vi "M100DailyOutputAutoNew.vi"() -> ()   [LabVIEW 2012]
uses:
  <vilib>/Utility/NIReport.llb/NI_report.lvclass
  <vilib>/addons/database/Connection.llb/DB Tools Open Connec (Path).vi
  <vilib>/addons/database/Connection.llb/Conn Execute.vi
  <vilib>/addons/database/Recordset.llb/Rec Fetch Recordset Data (R).vi
  <vilib>/addons/database/Recordset.llb/Rec Destroy - Connection.vi
  <vilib>/Utility/NIReport.llb/Append Text Table to Report (wrap).vi
  <vilib>/addons/database/_DB Variant To Data/Database Variant To Data.xnode
  <vilib>/addons/database/NI_Database_API.lvlib
  <vilib>/Utility/SMTP/NI_SMTPEmail.lvlib
  <vilib>/Utility/NIReport.llb/Excel/NI_Excel.lvclass
  <vilib>/addons/_office/NI_ReportGenerationToolkit.lvlib
panel:
  in  "Table Control 3":string[][](table)
  out "error out 4":errorcluster
  in  "Table Control 2":string[][](table)
  out "error out 3":errorcluster
  in  "Table Control":string[][](table)
  out "error out 2":errorcluster
  in  "Report Template":path=path "O:/Monitor/Report/M100DailyOutput.xls"
  out "error out":errorcluster
  out "spreadsheet string":string
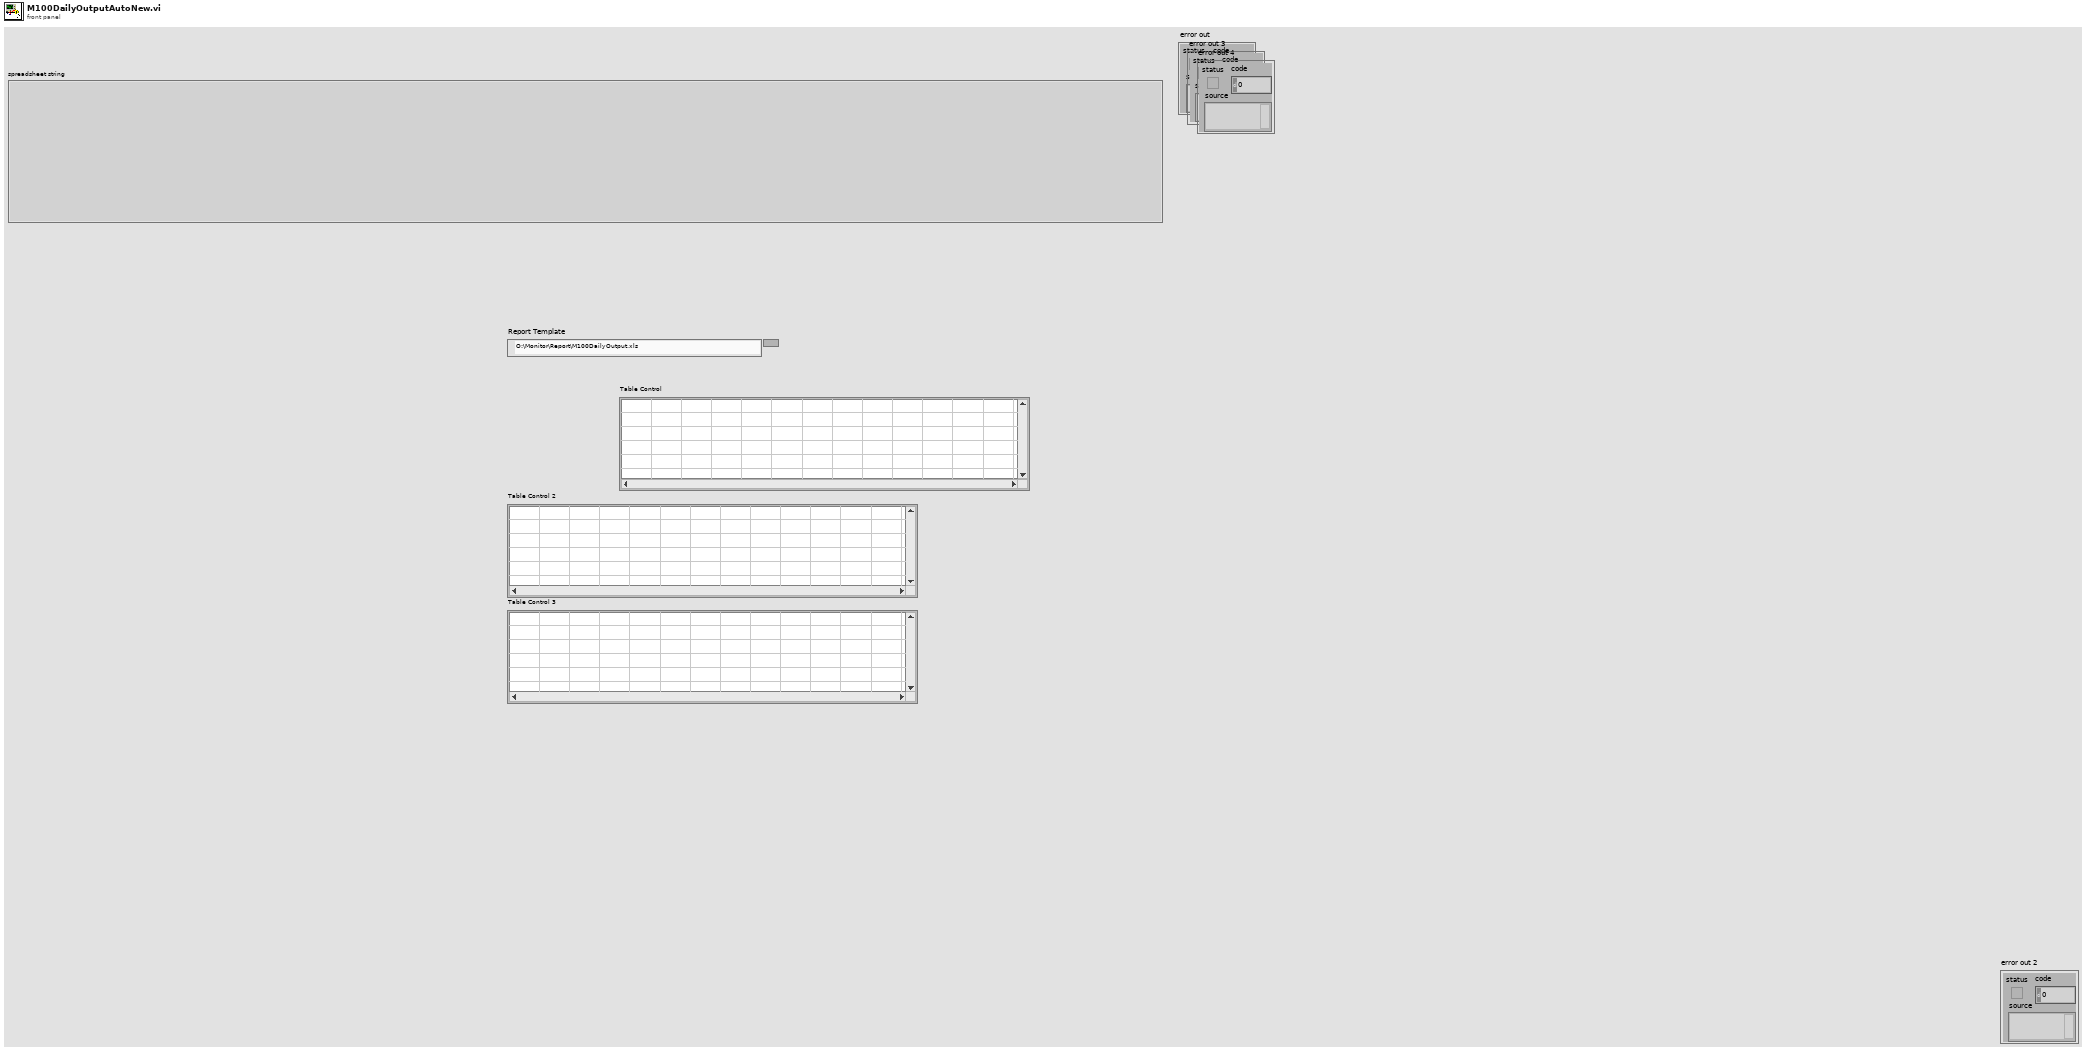
[diagram p1: front panel]
types:
  T1 = typedef "NI_Database_API.lvlib/Conn ObjectReference.ctl" = refnum<k1>
  T2 = typedef "NI_Database_API.lvlib/Rec ObjectReference.ctl" = refnum<k1>
  T3 = enum16{"Standard Report", "HTML", "Word", "Excel"}
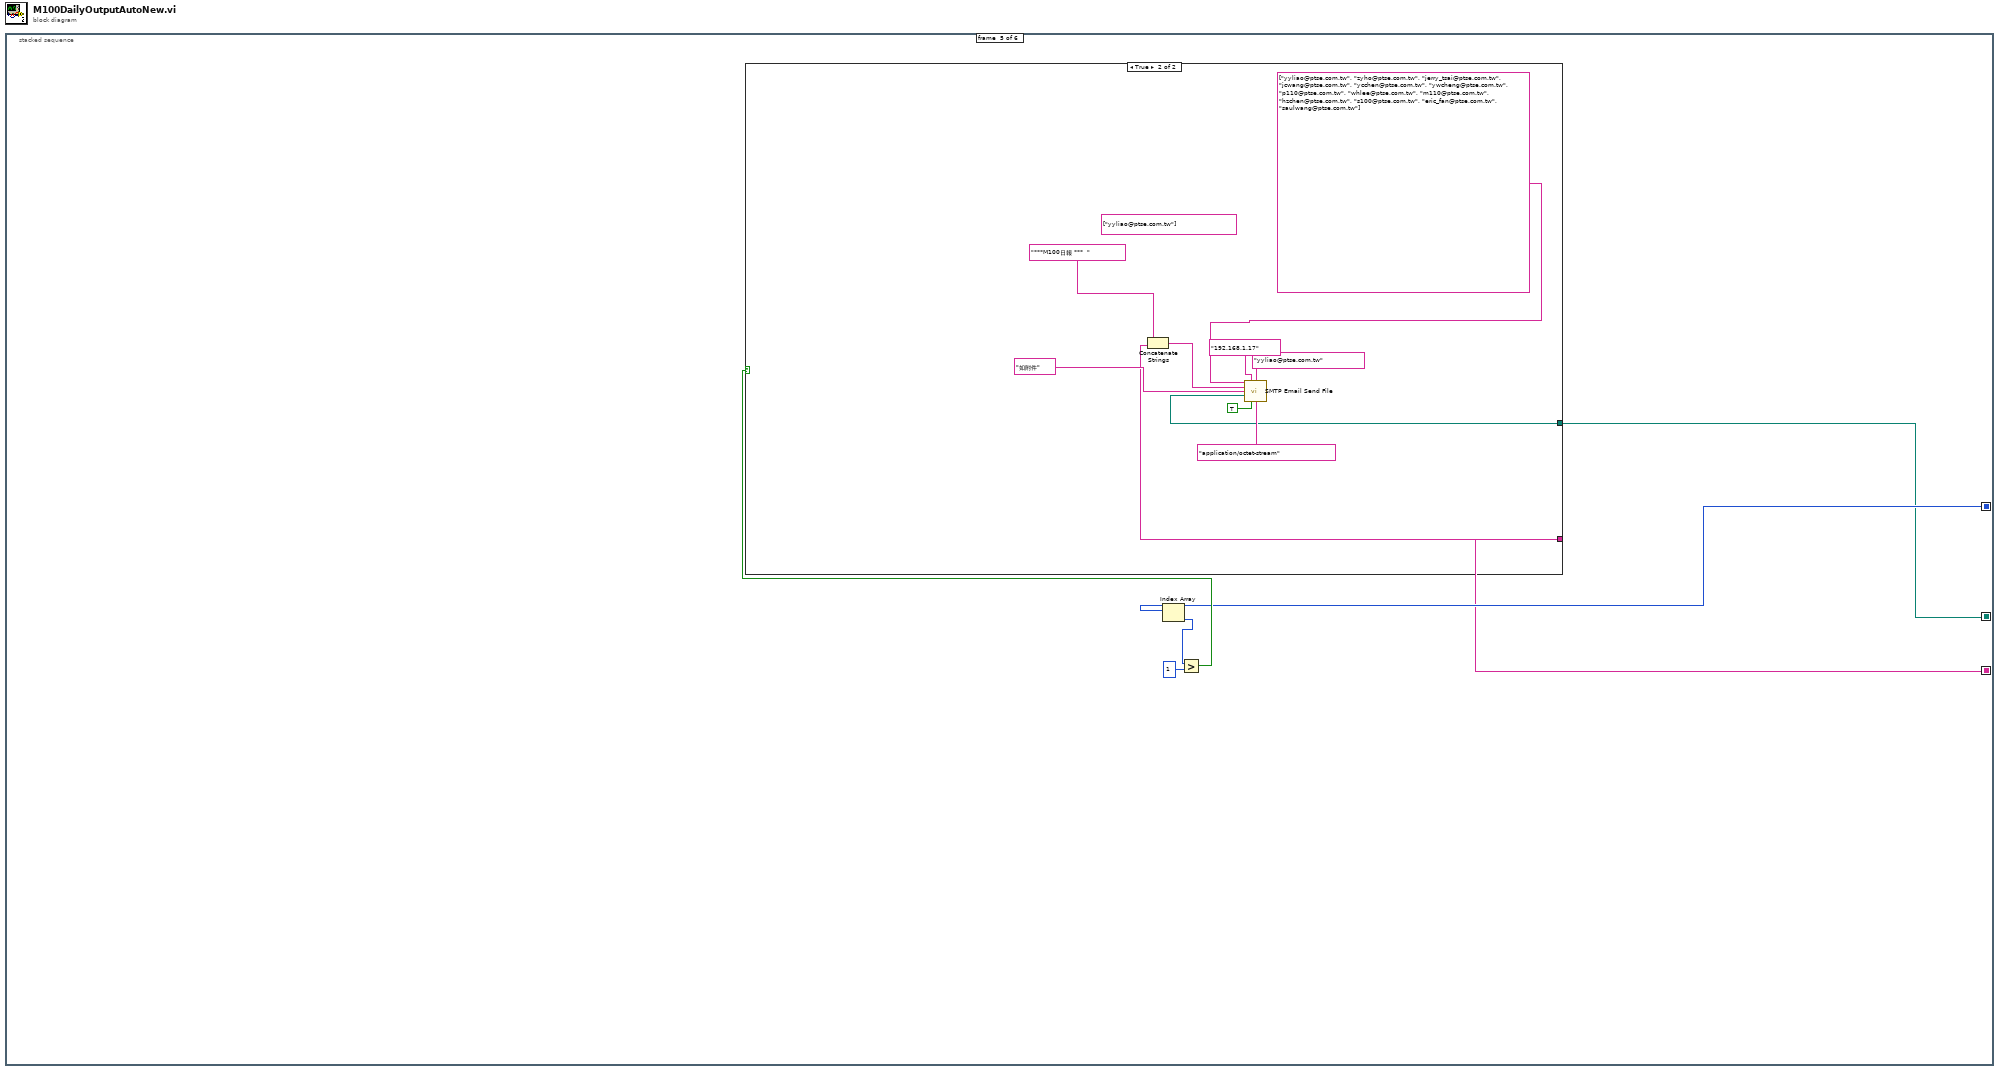
[diagram p0: block diagram]
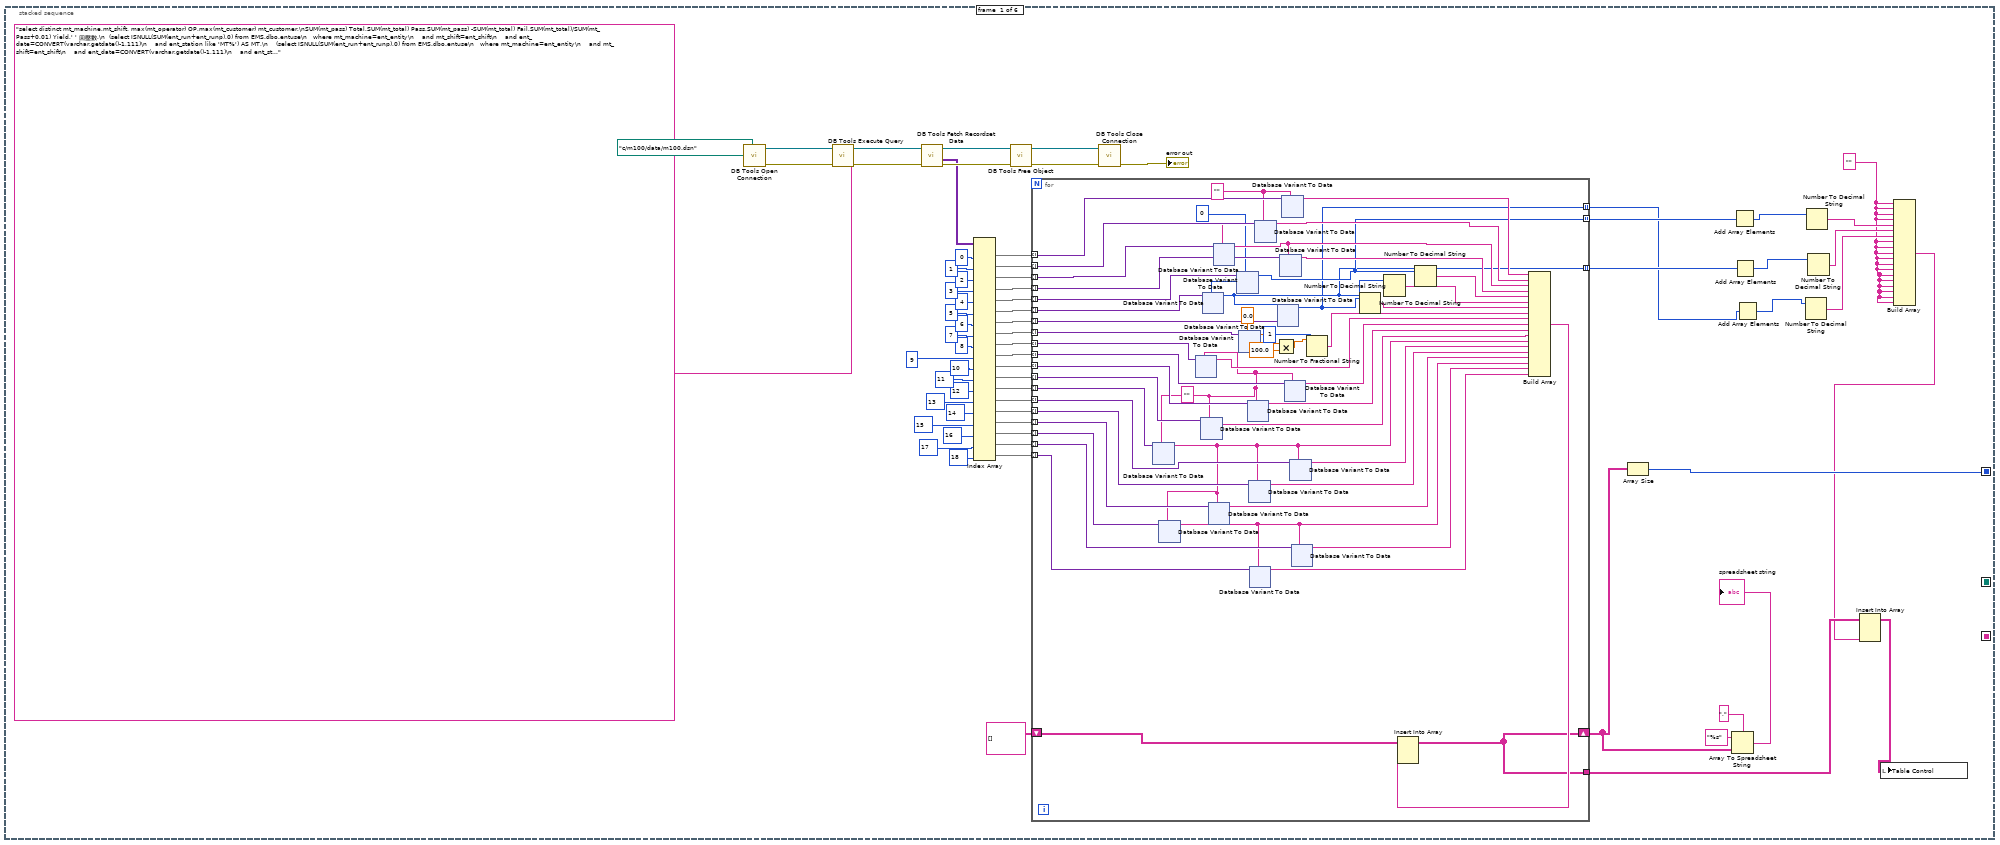
[diagram p2: hidden frame]
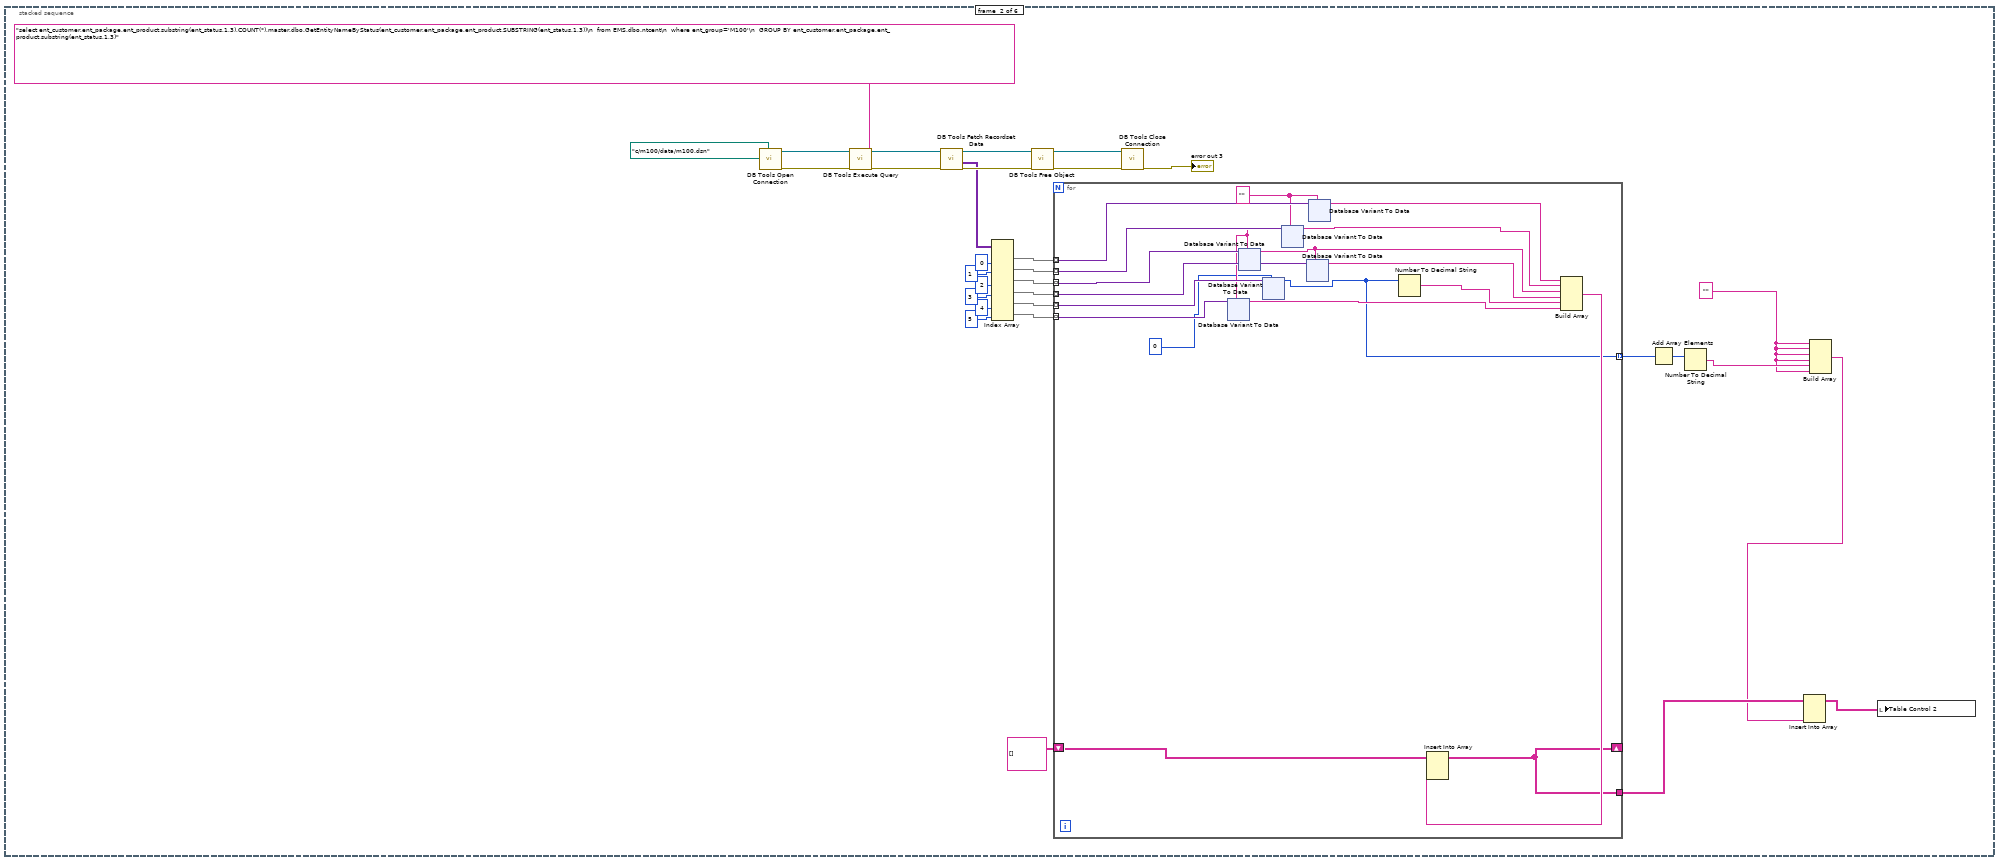
[diagram p3: hidden frame]
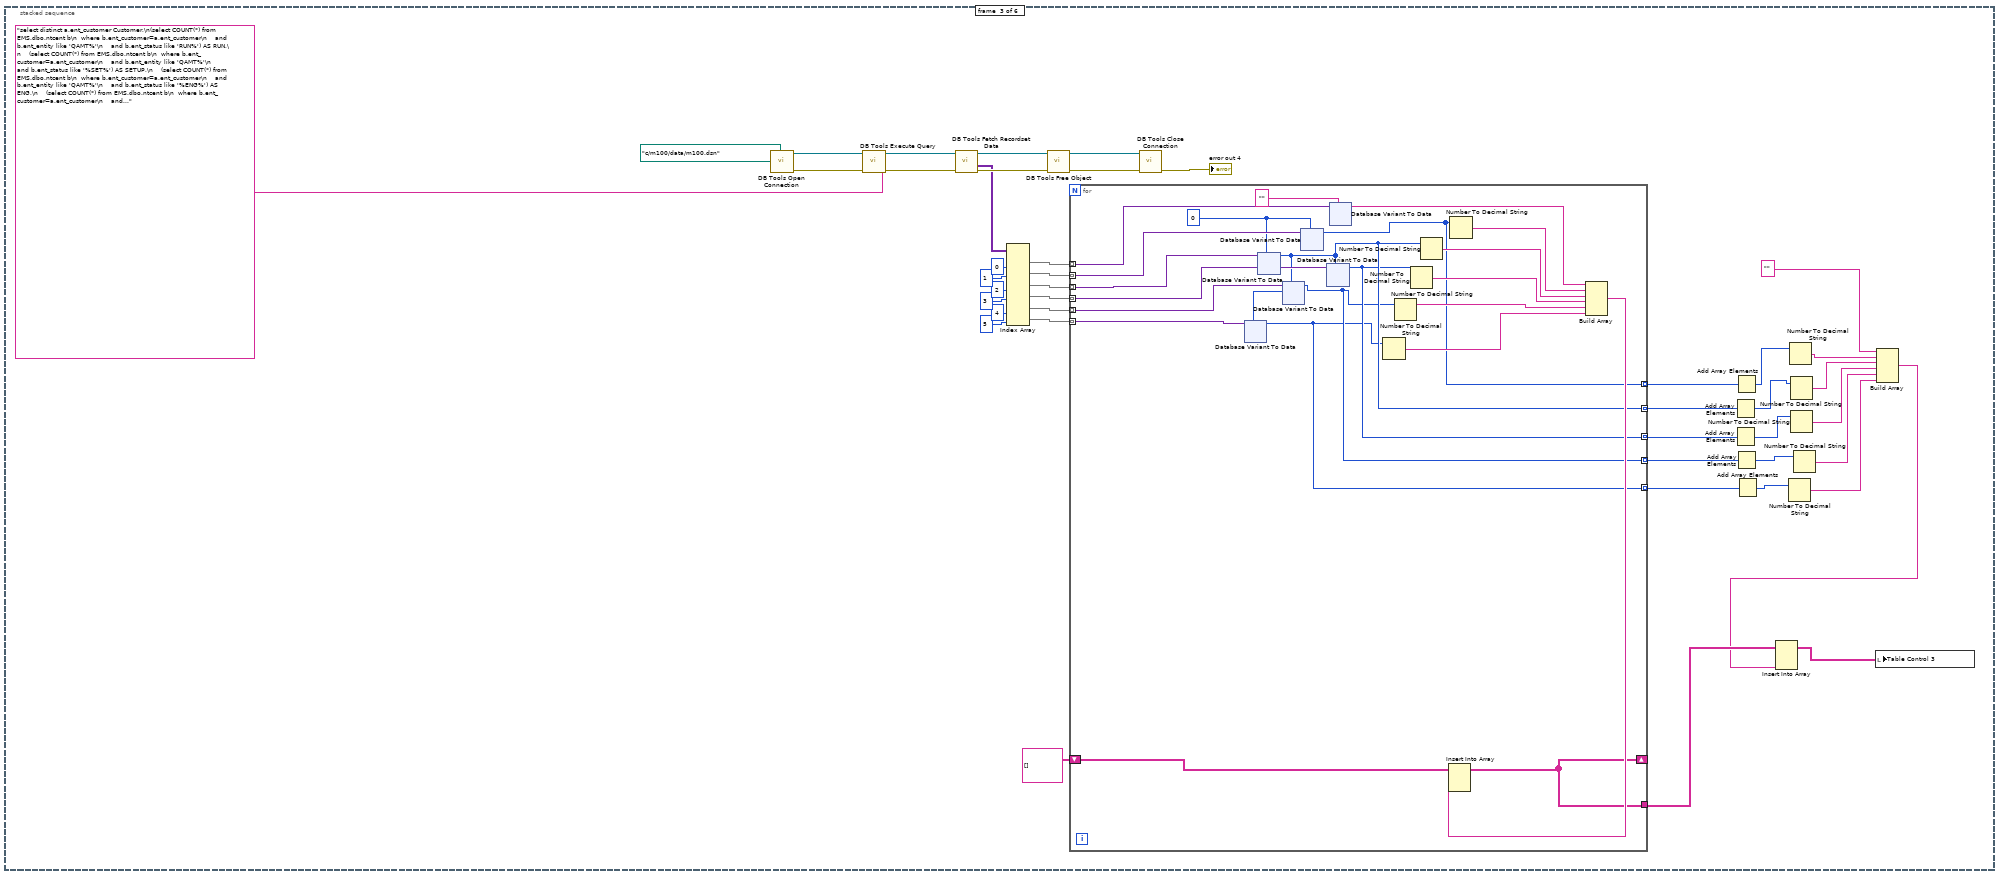
[diagram p4: hidden frame]
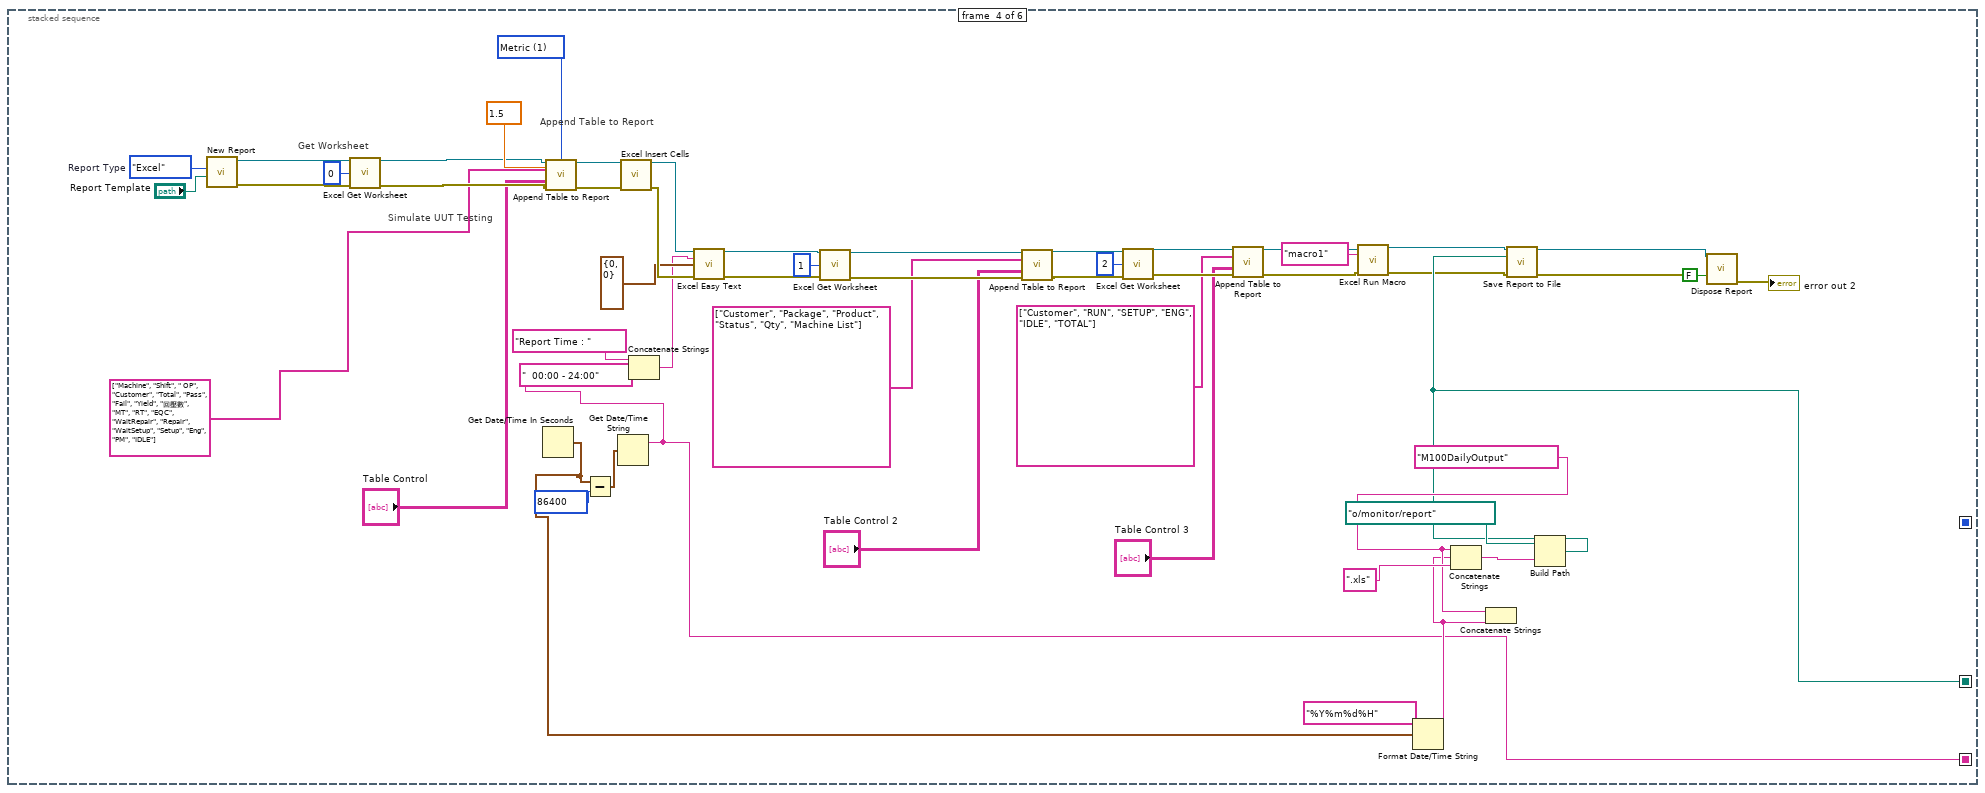
[diagram p5: hidden frame]
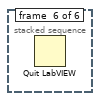
[diagram p7: hidden frame]
diagram:
  n1 = stacked-sequence {
    seq-local: [w37 _ _ _ _ _] -> [_ _ _ _ w1285 _]
    seq-local: [_ _ _ w1251 _ _] -> [_ _ _ _ w1284 _]
    seq-local: [_ _ _ w1250 _ _] -> [_ _ _ _ w1283 _]
    frame #0 {
      w4 = ""
      n2 = call-poly <vilib>:"DB Tools Open Connection.vi"("connection information"=path "c:/m100/data/m100.dsn") -> ("error out"=w64:errorcluster, "connection reference"=w68:T1)  [unwired: 7 in]
      n3 = call-poly <vilib>:"DB Tools Execute Query.vi"("error in (no error)"=w64, "SQL query"="select distinct mt_machine,mt_shift, max(mt_operator) OP,max(mt_customer) mt_customer,\nSUM(mt_pass) Total,SUM(mt_total) Pass,SUM(mt_pass) -SUM(mt_total) Fail,SUM(mt_total)/SUM(mt_Pass+0.01) Yield,' ' 回壓數,\n  (select ISNULL(SUM(ent_run+ent_runp),0) from EMS.dbo.entuse\n   where mt_machine=ent_entity\n    and mt_shift=ent_shift\n    and ent_date=CONVERT(varchar,getdate()-1,111)\n    and ent_station like 'MT%') AS MT,\n    (select ISNULL(SUM(ent_run+ent_runp),0) from EMS.dbo.entuse\n   where mt_machine=ent_entity\n    and mt_shift=ent_shift\n    and ent_date=CONVERT(varchar,getdate()-1,111)\n    and ent_station like 'RT%') AS RT,\n    (select ISNULL(SUM(ent_run+ent_runp),0) from EMS.dbo.entuse\n   where mt_machine=ent_entity\n    and mt_shift=ent_shift\n    and ent_date=CONVERT(varchar,getdate()-1,111)\n    and ent_station like 'EQ%') AS EQC,\n    (select ISNULL(SUM(ent_wait_repair),0) from EMS.dbo.entuse\n   where mt_machine=ent_entity\n    and mt_shift=ent_shift\n    and ent_date=CONVERT(varchar,getdate()-1,111)) as WaitRepair,\n     (select ISNULL(SUM(ent_repair),0) from EMS.dbo.entuse\n   where mt_machine=ent_entity\n    and mt_shift=ent_shift\n    and ent_date=CONVERT(varchar,getdate()-1,111)) as Repair,\n    (select ISNULL(SUM(ent_wait_setup),0) from EMS.dbo.entuse\n   where mt_machine=ent_entity\n    and mt_shift=ent_shift\n    and ent_date=CONVERT(varchar,getdate()-1,111)) as WaitSetup,\n     (select ISNULL(SUM(ent_setup),0) from EMS.dbo.entuse\n   where mt_machine=ent_entity\n    and mt_shift=ent_shift\n    and ent_date=CONVERT(varchar,getdate()-1,111)) as Setup,\n    (select ISNULL(SUM(ent_eng),0) from EMS.dbo.entuse\n   where mt_machine=ent_entity\n    and mt_shift=ent_shift\n    and ent_date=CONVERT(varchar,getdate()-1,111)) as Eng,\n     (select ISNULL(SUM(ent_pm),0) from EMS.dbo.entuse\n   where mt_machine=ent_entity\n    and mt_shift=ent_shift\n    and ent_date=CONVERT(varchar,getdate()-1,111)) as PM,\n    (select ISNULL(SUM(ent_idle),0) from EMS.dbo.entuse\n   where mt_machine=ent_entity\n    and mt_shift=ent_shift\n    and ent_date=CONVERT(varchar,getdate()-1,111)) as IDLE\n  from m100.dbo.mt_data\n  where CONVERT(varchar,mt_end,111)=CONVERT(varchar,getdate()-1,111)\n    and mt_machine like 'QAMT%'\n  group by mt_machine,mt_shift\n  order by mt_machine,mt_shift desc", "connection reference"=w68) -> ("error out"=w63:errorcluster, "recordset reference"=w67:T2)  [unwired: 5 in]
      n4 = call-poly <vilib>:"DB Tools Fetch Recordset Data.vi"("error in (no error)"=w63, "recordset reference"=w67) -> ("error out"=w62:errorcluster, "recordset data"=w31:variant[][], "recordset reference out"=w66:T2)  [unwired: 3 in]
      n5 = Index Array(array=w31, index (col) #1=0 ("disabled index (col)"), index (col) #2=1 ("index (col)"), index (col) #3=2 ("index (col)"), index (col) #4=3 ("index (col)"), index (col) #5=4 ("index (col)"), index (col) #6=5 ("index (col)"), index (col) #7=6 ("index (col)"), index (col) #8=7 ("index (col)"), index (col) #9=8 ("index (col)"), index (col) #10=9 ("index (col)"), index (col) #11=10 ("index (col)"), index (col) #12=11 ("index (col)"), index (col) #13=12 ("index (col)"), index (col) #14=13 ("index (col)"), index (col) #15=14 ("index (col)"), index (col) #16=15 ("index (col)"), index (col) #17=16 ("index (col)"), index (col) #18=17 ("index (col)"), index (col) #19=18 ("index (col)")) -> (element #1=w48:variant[], element #2=w47:variant[], element #3=w46:variant[], element #4=w45:variant[], element #5=w44:variant[], element #6=w43:variant[], element #7=w42:variant[], element #8=w41:variant[], element #9=w40:variant[], element #10=w39:variant[], element #11=w38:variant[], element #12=w34:variant[], element #13=w33:variant[], element #14=w25:variant[], element #15=w24:variant[], element #16=w23:variant[], element #17=w22:variant[], element #18=w21:variant[], element #19=w15:variant[])  [unwired: 19 in]
      n6 = call-poly <vilib>:"DB Tools Free Object.vi"("error in (no error)"=w62, "recordset reference"=w66) -> ("error out"=w61:errorcluster, "connection reference"=w65:T1)  [unwired: 8 in]
      n7 = for {
        tunnel: w48 -> [w121] mode=indexing
        tunnel: w47 -> [w120] mode=indexing
        tunnel: w46 -> [w119] mode=indexing
        tunnel: w45 -> [w118] mode=indexing
        tunnel: w44 -> [w117] mode=indexing
        tunnel: w43 -> [w116] mode=indexing
        tunnel: w42 -> [w115] mode=indexing
        tunnel: w41 -> [w114] mode=indexing
        tunnel: w40 -> [w113] mode=indexing
        tunnel: w39 -> [w112] mode=indexing
        tunnel: w38 -> [w111] mode=indexing
        tunnel: [w108] -> w3
        shift-right: [w108] -> w17
        shift-left: string[][] [] -> [w107]
        tunnel: w34 -> [w106] mode=indexing
        tunnel: w33 -> [w105] mode=indexing
        tunnel: w25 -> [w96] mode=indexing
        tunnel: w24 -> [w95] mode=indexing
        tunnel: w23 -> [w94] mode=indexing
        tunnel: w22 -> [w93] mode=indexing
        tunnel: w21 -> [w92] mode=indexing
        tunnel: w15 -> [w86] mode=indexing
        tunnel: [w72] -> w10 mode=indexing
        tunnel: [w71] -> w9 mode=indexing
        tunnel: [w70] -> w8 mode=indexing
        w78 = 0
        w73 = ""
        w102 = ""
        n8 = xnode "Database Variant To Data"("database variant"=w105, "type"=w73) -> ("data"=w91:string)  [unwired: 1 in, 1 out]
        n9 = xnode "Database Variant To Data"("database variant"=w93, "type"=w91) -> ("data"=w85:string)  [unwired: 1 in, 1 out]
        n10 = xnode "Database Variant To Data"("database variant"=w113, "type"=w73) -> ("data"=w99:string)  [unwired: 1 in, 1 out]
        n11 = xnode "Database Variant To Data"("database variant"=w106, "type"=w73) -> ("data"=w104:string)  [unwired: 1 in, 1 out]
        n12 = xnode "Database Variant To Data"("database variant"=w116, "type"=w78) -> ("data"=w71:i32)  [unwired: 1 in, 1 out]
        n13 = xnode "Database Variant To Data"("database variant"=w94, "type"=w91) -> ("data"=w88:string)  [unwired: 1 in, 1 out]
        n14 = xnode "Database Variant To Data"("database variant"=w119, "type"=w102) -> ("data"=w100:string)  [unwired: 1 in, 1 out]
        n15 = xnode "Database Variant To Data"("database variant"=w117, "type"=w78) -> ("data"=w72:i32)  [unwired: 1 in, 1 out]
        n16 = xnode "Database Variant To Data"("database variant"=w114, "type"=0.0) -> ("data"=w82:dbl)  [unwired: 1 in, 1 out]
        n17 = xnode "Database Variant To Data"("database variant"=w111, "type"=w73) -> ("data"=w97:string)  [unwired: 1 in, 1 out]
        n18 = xnode "Database Variant To Data"("database variant"=w95, "type"=w91) -> ("data"=w89:string)  [unwired: 1 in, 1 out]
        n19 = xnode "Database Variant To Data"("database variant"=w86, "type"=w85) -> ("data"=w84:string)  [unwired: 1 in, 1 out]
        n20 = xnode "Database Variant To Data"("database variant"=w120, "type"=w102) -> ("data"=w103:string)  [unwired: 1 in, 1 out]
        n21 = Multiply(x=w82, y=100.0) -> (x*y=w80:dbl)
        n22 = xnode "Database Variant To Data"("database variant"=w115, "type"=w71) -> ("data"=w70:i32)  [unwired: 1 in, 1 out]
        n23 = xnode "Database Variant To Data"("database variant"=w118, "type"=w100) -> ("data"=w101:string)  [unwired: 1 in, 1 out]
        n24 = xnode "Database Variant To Data"("database variant"=w121, "type"=w102) -> ("data"=w110:string)  [unwired: 1 in, 1 out]
        n25 = xnode "Database Variant To Data"("database variant"=w112, "type"=w73) -> ("data"=w98:string)  [unwired: 1 in, 1 out]
        n26 = xnode "Database Variant To Data"("database variant"=w96, "type"=w91) -> ("data"=w90:string)  [unwired: 1 in, 1 out]
        n27 = xnode "Database Variant To Data"("database variant"=w92, "type"=w85) -> ("data"=w87:string)  [unwired: 1 in, 1 out]
        n28 = Number To Fractional String(number=w80, precision (6)=i16 1) -> (F-format string=w75:string)  [unwired: 2 in]
        n29 = Number To Decimal String(number=w70) -> (decimal integer string=w74:string)  [unwired: 1 in]
        n30 = Number To Decimal String(number=w71) -> (decimal integer string=w76:string)  [unwired: 1 in]
        n31 = Number To Decimal String(number=w72) -> (decimal integer string=w77:string)  [unwired: 1 in]
        n32 = Build Array(w110, w103, w100, w101, w77, w76, w74, w75, w99, w98, w97, w104, w91, w90, w89, w88, w85, w87, w84) -> (w109:string[])
        n33 = Insert Into Array(array=w107, new element=w109) -> (w108:string[][])  [unwired: 2 in]
      }
      n34 = call <vilib>:"DB Tools Close Connection.vi"("error in (no error)"=w61, "connection reference"=w65) -> ("error out"=→"error out":errorcluster)  [unwired: 5 in]
      n35 = Array Size(array=w17) -> (size(s)=w37:i32[])
      n36 = Array To Spreadsheet String(delimiter (Tab)=",", array=w17, 3:"%s" ("format string")) -> (spreadsheet string=→"spreadsheet string":string)
      n37 = Add Array Elements(numeric array=w10) -> (sum=w13:i32)
      n38 = Add Array Elements(numeric array=w9) -> (sum=w12:i32)
      n39 = Add Array Elements(numeric array=w8) -> (sum=w11:i32)
      n40 = Number To Decimal String(number=w11) -> (decimal integer string=w5:string)  [unwired: 1 in]
      n41 = Number To Decimal String(number=w13) -> (decimal integer string=w7:string)  [unwired: 1 in]
      n42 = Number To Decimal String(number=w12) -> (decimal integer string=w6:string)  [unwired: 1 in]
      n43 = Build Array(w4, w4, w4, w4, w7, w6, w5, w4, w4, w4, w4, w4, w4, w4, w4, w4, w4, w4, w4) -> (w2:string[])
      n44 = Insert Into Array(array=w3, new element=w2) -> (w1:string[][])  [unwired: 2 in]
      n45 = local write "Table Control"(w1) -> ()
    }
    frame #1 {
      w731 = ""
      n46 = call-poly <vilib>:"DB Tools Open Connection.vi"("connection information"=path "c:/m100/data/m100.dsn") -> ("error out"=w756:errorcluster, "connection reference"=w760:T1)  [unwired: 7 in]
      n47 = call-poly <vilib>:"DB Tools Execute Query.vi"("error in (no error)"=w756, "SQL query"="select ent_customer,ent_package,ent_product,substring(ent_status,1,3),COUNT(*),master.dbo.GetEntityNameByStatus(ent_customer,ent_package,ent_product,SUBSTRING(ent_status,1,3))\n  from EMS.dbo.ntcent\n  where ent_group='M100'\n  GROUP BY ent_customer,ent_package,ent_product,substring(ent_status,1,3)", "connection reference"=w760) -> ("error out"=w755:errorcluster, "recordset reference"=w759:T2)  [unwired: 5 in]
      n48 = call-poly <vilib>:"DB Tools Fetch Recordset Data.vi"("error in (no error)"=w755, "recordset reference"=w759) -> ("error out"=w754:errorcluster, "recordset data"=w738:variant[][], "recordset reference out"=w758:T2)  [unwired: 3 in]
      n49 = Index Array(array=w738, index (col) #1=0 ("disabled index (col)"), index (col) #2=1 ("index (col)"), index (col) #3=2 ("index (col)"), index (col) #4=3 ("index (col)"), index (col) #5=4 ("index (col)"), index (col) #6=5 ("index (col)")) -> (element #1=w745:variant[], element #2=w744:variant[], element #3=w743:variant[], element #4=w742:variant[], element #5=w741:variant[], element #6=w740:variant[])  [unwired: 6 in]
      n50 = call-poly <vilib>:"DB Tools Free Object.vi"("error in (no error)"=w754, "recordset reference"=w758) -> ("error out"=w753:errorcluster, "connection reference"=w757:T1)  [unwired: 8 in]
      n51 = for {
        tunnel: w745 -> [w779] mode=indexing
        tunnel: w744 -> [w778] mode=indexing
        tunnel: w743 -> [w777] mode=indexing
        tunnel: w742 -> [w776] mode=indexing
        tunnel: w741 -> [w775] mode=indexing
        tunnel: w740 -> [w774] mode=indexing
        tunnel: [w771] -> w734
        shift-right: [w771] -> _
        shift-left: string[][] [] -> [w770]
        tunnel: [w762] -> w736 mode=indexing
        w765 = ""
        n52 = xnode "Database Variant To Data"("database variant"=w774, "type"=w765) -> ("data"=w766:string)  [unwired: 1 in, 1 out]
        n53 = xnode "Database Variant To Data"("database variant"=w777, "type"=w765) -> ("data"=w767:string)  [unwired: 1 in, 1 out]
        n54 = xnode "Database Variant To Data"("database variant"=w775, "type"=0) -> ("data"=w762:i32)  [unwired: 1 in, 1 out]
        n55 = xnode "Database Variant To Data"("database variant"=w778, "type"=w765) -> ("data"=w769:string)  [unwired: 1 in, 1 out]
        n56 = xnode "Database Variant To Data"("database variant"=w776, "type"=w767) -> ("data"=w768:string)  [unwired: 1 in, 1 out]
        n57 = xnode "Database Variant To Data"("database variant"=w779, "type"=w765) -> ("data"=w773:string)  [unwired: 1 in, 1 out]
        n58 = Number To Decimal String(number=w762) -> (decimal integer string=w763:string)  [unwired: 1 in]
        n59 = Build Array(w773, w769, w767, w768, w763, w766) -> (w772:string[])
        n60 = Insert Into Array(array=w770, new element=w772) -> (w771:string[][])  [unwired: 2 in]
      }
      n61 = call <vilib>:"DB Tools Close Connection.vi"("error in (no error)"=w753, "connection reference"=w757) -> ("error out"=→"error out 3":errorcluster)  [unwired: 5 in]
      n62 = Add Array Elements(numeric array=w736) -> (sum=w735:i32)
      n63 = Number To Decimal String(number=w735) -> (decimal integer string=w732:string)  [unwired: 1 in]
      n64 = Build Array(w731, w731, w731, w731, w732, w731) -> (w730:string[])
      n65 = Insert Into Array(array=w734, new element=w730) -> (w733:string[][])  [unwired: 2 in]
      n66 = local write "Table Control 2"(w733) -> ()
    }
    frame #2 {
      n67 = call-poly <vilib>:"DB Tools Open Connection.vi"("connection information"=path "c:/m100/data/m100.dsn") -> ("error out"=w1010:errorcluster, "connection reference"=w1014:T1)  [unwired: 7 in]
      n68 = call-poly <vilib>:"DB Tools Execute Query.vi"("error in (no error)"=w1010, "SQL query"="select distinct a.ent_customer Customer,\n(select COUNT(*) from EMS.dbo.ntcent b\n  where b.ent_customer=a.ent_customer\n    and b.ent_entity like 'QAMT%'\n    and b.ent_status like 'RUN%') AS RUN,\n    (select COUNT(*) from EMS.dbo.ntcent b\n  where b.ent_customer=a.ent_customer\n    and b.ent_entity like 'QAMT%'\n    and b.ent_status like '%SET%') AS SETUP,\n    (select COUNT(*) from EMS.dbo.ntcent b\n  where b.ent_customer=a.ent_customer\n    and b.ent_entity like 'QAMT%'\n    and b.ent_status like '%ENG%') AS ENG,\n    (select COUNT(*) from EMS.dbo.ntcent b\n  where b.ent_customer=a.ent_customer\n    and b.ent_entity like 'QAMT%'\n    and b.ent_status like '%IDLE%') AS IDLE,\n    (select COUNT(*) from EMS.dbo.ntcent b\n  where b.ent_customer=a.ent_customer\n    and b.ent_entity like 'QAMT%'\n    ) AS TOTAL\n    FROM EMS.dbo.ntcent a\n    where a.ent_entity like 'QAMT%'", "connection reference"=w1014) -> ("error out"=w1009:errorcluster, "recordset reference"=w1013:T2)  [unwired: 5 in]
      n69 = call-poly <vilib>:"DB Tools Fetch Recordset Data.vi"("error in (no error)"=w1009, "recordset reference"=w1013) -> ("error out"=w1008:errorcluster, "recordset data"=w992:variant[][], "recordset reference out"=w1012:T2)  [unwired: 3 in]
      n70 = Index Array(array=w992, index (col) #1=0 ("disabled index (col)"), index (col) #2=1 ("index (col)"), index (col) #3=2 ("index (col)"), index (col) #4=3 ("index (col)"), index (col) #5=4 ("index (col)"), index (col) #6=5 ("index (col)")) -> (element #1=w999:variant[], element #2=w998:variant[], element #3=w997:variant[], element #4=w996:variant[], element #5=w995:variant[], element #6=w994:variant[])  [unwired: 6 in]
      n71 = call-poly <vilib>:"DB Tools Free Object.vi"("error in (no error)"=w1008, "recordset reference"=w1012) -> ("error out"=w1007:errorcluster, "connection reference"=w1011:T1)  [unwired: 8 in]
      n72 = for {
        tunnel: w999 -> [w1037] mode=indexing
        tunnel: w998 -> [w1036] mode=indexing
        tunnel: w997 -> [w1035] mode=indexing
        tunnel: w996 -> [w1034] mode=indexing
        tunnel: w995 -> [w1033] mode=indexing
        tunnel: w994 -> [w1032] mode=indexing
        tunnel: [w1029] -> w973
        shift-right: [w1029] -> _
        shift-left: string[][] [] -> [w1028]
        tunnel: [w1020] -> w990 mode=indexing
        tunnel: [w1019] -> w989 mode=indexing
        tunnel: [w1018] -> w988 mode=indexing
        tunnel: [w1017] -> w987 mode=indexing
        tunnel: [w1016] -> w986 mode=indexing
        w1026 = 0
        n73 = xnode "Database Variant To Data"("database variant"=w1035, "type"=w1026) -> ("data"=w1019:i32)  [unwired: 1 in, 1 out]
        n74 = xnode "Database Variant To Data"("database variant"=w1032, "type"=w1019) -> ("data"=w1016:i32)  [unwired: 1 in, 1 out]
        n75 = xnode "Database Variant To Data"("database variant"=w1033, "type"=w1019) -> ("data"=w1017:i32)  [unwired: 1 in, 1 out]
        n76 = xnode "Database Variant To Data"("database variant"=w1036, "type"=w1026) -> ("data"=w1020:i32)  [unwired: 1 in, 1 out]
        n77 = xnode "Database Variant To Data"("database variant"=w1034, "type"=w1019) -> ("data"=w1018:i32)  [unwired: 1 in, 1 out]
        n78 = xnode "Database Variant To Data"("database variant"=w1037, "type"="") -> ("data"=w1031:string)  [unwired: 1 in, 1 out]
        n79 = Number To Decimal String(number=w1016) -> (decimal integer string=w1021:string)  [unwired: 1 in]
        n80 = Number To Decimal String(number=w1017) -> (decimal integer string=w1022:string)  [unwired: 1 in]
        n81 = Number To Decimal String(number=w1018) -> (decimal integer string=w1023:string)  [unwired: 1 in]
        n82 = Number To Decimal String(number=w1019) -> (decimal integer string=w1024:string)  [unwired: 1 in]
        n83 = Number To Decimal String(number=w1020) -> (decimal integer string=w1025:string)  [unwired: 1 in]
        n84 = Build Array(w1031, w1025, w1024, w1023, w1022, w1021) -> (w1030:string[])
        n85 = Insert Into Array(array=w1028, new element=w1030) -> (w1029:string[][])  [unwired: 2 in]
      }
      n86 = call <vilib>:"DB Tools Close Connection.vi"("error in (no error)"=w1007, "connection reference"=w1011) -> ("error out"=→"error out 4":errorcluster)  [unwired: 5 in]
      n87 = Add Array Elements(numeric array=w989) -> (sum=w984:i32)
      n88 = Add Array Elements(numeric array=w988) -> (sum=w983:i32)
      n89 = Add Array Elements(numeric array=w990) -> (sum=w985:i32)
      n90 = Add Array Elements(numeric array=w987) -> (sum=w982:i32)
      n91 = Add Array Elements(numeric array=w986) -> (sum=w981:i32)
      n92 = Number To Decimal String(number=w981) -> (decimal integer string=w975:string)  [unwired: 1 in]
      n93 = Number To Decimal String(number=w985) -> (decimal integer string=w979:string)  [unwired: 1 in]
      n94 = Number To Decimal String(number=w984) -> (decimal integer string=w978:string)  [unwired: 1 in]
      n95 = Number To Decimal String(number=w983) -> (decimal integer string=w977:string)  [unwired: 1 in]
      n96 = Number To Decimal String(number=w982) -> (decimal integer string=w976:string)  [unwired: 1 in]
      n97 = Build Array("", w979, w978, w977, w976, w975) -> (w972:string[])
      n98 = Insert Into Array(array=w973, new element=w972) -> (w974:string[][])  [unwired: 2 in]
      n99 = local write "Table Control 3"(w974) -> ()
    }
    frame #3 {
      w1257 = u16 1 items=["US", "Metric", "Default"] ("measurement system")
      w1260 = "M100DailyOutput"
      w1282 = T3."Excel"  # Report Type
      # "Simulate UUT Testing"
      # "Append Table to Report"
      # "Get Worksheet"
      n100 = call <vilib>:"New Report.vi"("report type"=w1282, "template (empty)"="Report Template") -> ("report out"=w1277:refnum<class "NI_report.lvclass">, "error out"=w1276:errorcluster)  [unwired: 12 in]
      n101 = call <vilib>:"Excel Get Worksheet.vi"("report in"=w1277, "worksheet index (0)"=0, "error in (no error)"=w1276) -> ("report out"=w1266:refnum<class "NI_report.lvclass">, "error out"=w1265:errorcluster)  [unwired: 11 in]
      n102 = Get Date/Time In Seconds() -> (seconds since 1Jan1904=w1254:timestamp)
      n103 = call-poly <vilib>:"Append Table to Report.vi"("report in"=w1266, "column width (1)"=1.5, "measurement system"=w1257, "column headers"=string[] ["Machine", "Shift", " OP", "Customer", "Total", "Pass", "Fail", "Yield", "回壓數", "MT", "RT", "EQC", "WaitRepair", "Repair", "WaitSetup", "Setup", "Eng", "PM", "IDLE"] ("Array"), "text data"="Table Control", "error in (no error)"=w1265) -> ("report out"=w1279:refnum<class "NI_report.lvclass">, "error out"=w1278:errorcluster)  [unwired: 6 in, 2 out]
      n104 = Subtract(x=w1254, y=86400) -> (x-y=w1258:timestamp)
      n105 = Get Date/Time String(seconds (now)=w1258) -> (date string=w1250:string)  [unwired: 2 in, 1 out]
      n106 = call <vilib>:"Excel Insert Cells.vi"("report in"=w1279, "error in (no error)"=w1278) -> ("report out"=w1273:refnum<class "NI_report.lvclass">, "error out"=w1272:errorcluster)  [unwired: 12 in]
      n107 = Concatenate Strings("Report Time : " ("string"), w1250, "  00:00 - 24:00" ("string")) -> (w1269:string)
      n108 = call <vilib>:"Excel Easy Text.vi"("report in"=w1273, "text"=w1269, "start (-1, -1)"=cluster{"row":i32, "column":i32} {"row"=0, "column"=0} ("end (-1, -1)"), "error in (no error)"=w1272) -> ("report out"=w1248:refnum<class "NI_report.lvclass">, "error out"=w1247:errorcluster)  [unwired: 7 in, 3 out]
      n109 = call <vilib>:"Excel Get Worksheet.vi"("report in"=w1248, "worksheet index (0)"=1, "error in (no error)"=w1247) -> ("report out"=w1245:refnum<class "NI_report.lvclass">, "error out"=w1244:errorcluster)  [unwired: 11 in]
      n110 = call-poly <vilib>:"Append Table to Report.vi"("report in"=w1245, "column headers"=string[] ["Customer", "Package", "Product", "Status", "Qty", "Machine List"], "text data"="Table Control 2", "error in (no error)"=w1244) -> ("report out"=w1241:refnum<class "NI_report.lvclass">, "error out"=w1240:errorcluster)  [unwired: 8 in, 2 out]
      n111 = call <vilib>:"Excel Get Worksheet.vi"("report in"=w1241, "worksheet index (0)"=2, "error in (no error)"=w1240) -> ("report out"=w1239:refnum<class "NI_report.lvclass">, "error out"=w1238:errorcluster)  [unwired: 11 in]
      n112 = call-poly <vilib>:"Append Table to Report.vi"("report in"=w1239, "column headers"=string[] ["Customer", "RUN", "SETUP", "ENG", "IDLE", "TOTAL"], "text data"="Table Control 3", "error in (no error)"=w1238) -> ("report out"=w1234:refnum<class "NI_report.lvclass">, "error out"=w1232:errorcluster)  [unwired: 8 in, 2 out]
      n113 = call <vilib>:"Excel Run Macro.vi"("report in"=w1234, "macro name"="macro1", "error in (no error)"=w1232) -> ("report out"=w1233:refnum<class "NI_report.lvclass">, "error out"=w1231:errorcluster)  [unwired: 10 in, 1 out]
      n114 = Format Date/Time String(time format string (%c)="%Y%m%d%H", seconds (now)=w1254) -> (date/time string=w1255:string)  [unwired: 1 in]
      n115 = Concatenate Strings(w1260, w1255, ".xls" ("string")) -> (w1261:string)
      n116 = Concatenate Strings(w1260, w1255) -> ()  [unwired: 1 out]
      n117 = Build Path(base path=path "o:/monitor/report", name or relative path=w1261) -> (appended path=w1251:path)
      n118 = call-dynamic "Save Report to File.vi"("report in"=w1233, "report file path"=w1251, "error in (no error)"=w1231) -> ("report out"=w1268:refnum<class "NI_report.lvclass">, "error out"=w1267:errorcluster)  [unwired: 11 in]
      n119 = call-dynamic "Dispose Report.vi"("report in"=w1268, "save changes? (F)"=FALSE, "error in (no error)"=w1267) -> ("error out"=→"error out 2":errorcluster)  [unwired: 12 in]
    }
    frame #4 {
      n120 = Index Array(array=w1285) -> (element=w1288:i32)  [unwired: 1 in]
      n121 = Greater?(x=w1288, y=1) -> (0:w1286:bool)
      n122 = case shown="True" w1286 {
        tunnel: w1284 -> [_ w1293]
        tunnel: w1283 -> [_ w1290]
        frame False {
        }
        frame True {
          (unwired) string[] ["yyliao@ptse.com.tw"] ("recipients")
          n123 = Concatenate Strings("***M100日報 ***  " ("subject ([No Subject])"), w1290) -> (w1291:string)
          n124 = call <vilib>:"SMTP Email Send File.vi"("recipients"=string[] ["yyliao@ptse.com.tw", "zyho@ptse.com.tw", "jerry_tsai@ptse.com.tw", "jcwang@ptse.com.tw", "ycchen@ptse.com.tw", "ywcheng@ptse.com.tw", "p110@ptse.com.tw", "whlee@ptse.com.tw", "m110@ptse.com.tw", "hzchen@ptse.com.tw", "s100@ptse.com.tw", "eric_fan@ptse.com.tw", "saulwang@ptse.com.tw"], "mail server"="192.168.1.17", "return address"="yyliao@ptse.com.tw", "subject ([No Subject])"=w1291, "message"="如附件", "file path"=w1293, "binary? (F)"=TRUE, "MIME content-type (application/octet-stream)"="application/octet-stream") -> ()  [unwired: 6 in, 2 out]
        }
      }
    }
    frame #5 {
      n125 = Quit LabVIEW() -> ()  [unwired: 1 in]
    }
  }
